vi "ParseI2CRHTempData.vi"(8 "error in (no error)":errorcluster, 11 "ByteArrayRecieved":u8[](array[numeric])) -> (0 "error out":errorcluster, 2 "Numeric":dbl, 3 "Numeric 2":dbl)   [LabVIEW 2019]
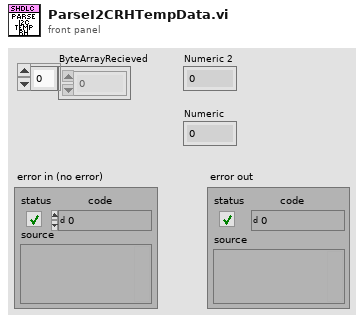
[diagram p1: front panel]
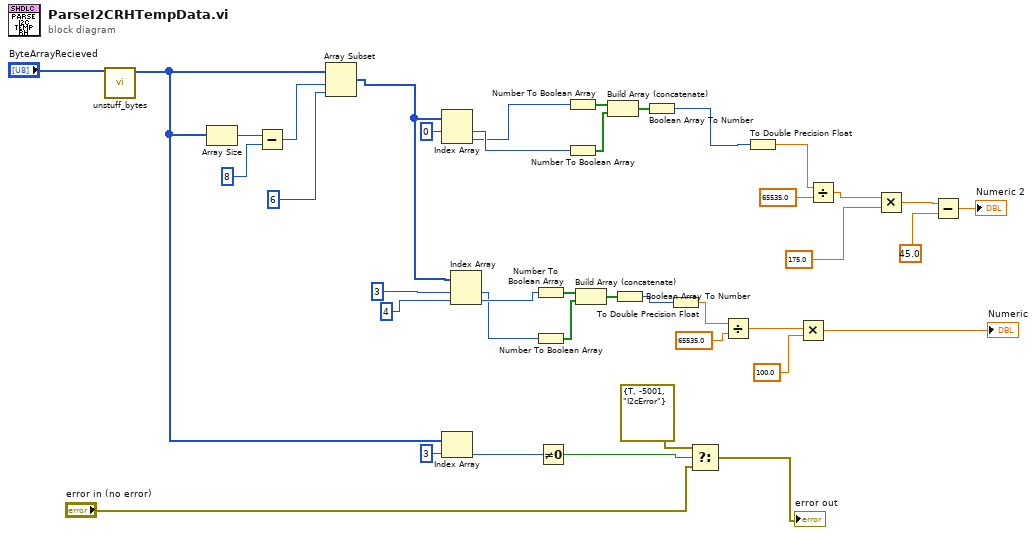
[diagram p0: block diagram]
diagram:
  n1 = call "unstuff_bytes.vi"("StuffedByteArrayIn"="ByteArrayRecieved") -> ("UnstuffedDataOut"=w3:u8[])  [unwired: 10 in]
  n2 = Array Size(array=w3) -> (size(s)=w9:i32)
  n3 = Subtract(x=w9, y=8) -> (x-y=w11:i32)
  n4 = Array Subset(array=w3, index=w11, length=6) -> (w8:u8[])
  n5 = Index Array(array=w8, index #1=0 ("index")) -> (element #1=w26:u8, element #2=w25:u8)  [unwired: 1 in]
  n6 = Index Array(array=w3, index=3) -> (element=w2:u8)
  n7 = Index Array(array=w8, index #1=3 ("index"), index #2=4 ("index")) -> (element #1=w32:u8, element #2=w33:u8)
  n8 = Number To Boolean Array(number=w33) -> (Boolean array=w29:bool[])
  n9 = Number To Boolean Array(number=w32) -> (Boolean array=w28:bool[])
  n10 = Not Equal To 0?(x=w2) -> (x != 0?=w1:bool)
  n11 = Number To Boolean Array(number=w25) -> (Boolean array=w14:bool[])
  n12 = Number To Boolean Array(number=w26) -> (Boolean array=w15:bool[])
  n13 = Build Array (concatenate)(w29, w28) -> (w27:bool[])
  n14 = Build Array (concatenate)(w14, w15) -> (w16:bool[])
  n15 = Boolean Array To Number(Boolean array=w27) -> (number=w34:u32)
  n16 = Boolean Array To Number(Boolean array=w16) -> (number=w17:u32)
  n17 = To Double Precision Float(number=w34) -> (double precision float=w35:dbl)
  n18 = Select(t=errorcluster {"status"=TRUE, "code"=-5001, "source"="I2cError"}, s=w1, f="error in (no error)") -> (s? t:f=→"error out":errorcluster)
  n19 = Divide(x=w35, y=65535.0) -> (x/y=w37:dbl)
  n20 = To Double Precision Float(number=w17) -> (double precision float=w19:dbl)
  n21 = Multiply(x=w37, y=100.0) -> (x*y=→"Numeric":dbl)
  n22 = Divide(x=w19, y=65535.0) -> (x/y=w20:dbl)
  n23 = Multiply(x=w20, y=175.0) -> (x*y=w22:dbl)
  n24 = Subtract(x=w22, y=45.0) -> (x-y=→"Numeric 2":dbl)
